vi "set_properties_dialog.vi"(8 "Graph Range Min/Max":T1, 9 "Graph Properties In":T3, 10 "All Properties":T4, 11 "Plot IDs":i32[](array[numeric])) -> (1 "Graph Properties Out":T3, 2 "All Properties Out":T4)   [LabVIEW 2020, in "3DPC_SurfacePlot.xctl"]
uses:
  <vilib>/Native 3D Graph/xcontrol/3DPC_SurfacePlot.xctl
  <vilib>/Native 3D Graph/typedefs/all_non_graph_prop.ctl
  <vilib>/Native 3D Graph/typedefs/prop_plot_all_array.ctl
  <vilib>/Native 3D Graph/typedefs/prop_plot_all.ctl
  <vilib>/Native 3D Graph/typedefs/prop_plot_projection.ctl
  <vilib>/Native 3D Graph/typedefs/prop_plot_surface.ctl
  <vilib>/Native 3D Graph/typedefs/prop_plot_contour.ctl
  <vilib>/Native 3D Graph/typedefs/prop_plot_normal.ctl
  <vilib>/Native 3D Graph/typedefs/prop_plot_point_line.ctl
  <vilib>/Native 3D Graph/typedefs/prop_value_pair_all.ctl
  <vilib>/Native 3D Graph/typedefs/prop_value_pair_1d.ctl
  <vilib>/Native 3D Graph/typedefs/prop_axes_all.ctl
  <vilib>/Native 3D Graph/typedefs/prop_axes_grid.ctl
  <vilib>/Native 3D Graph/typedefs/prop_axes_ticks.ctl
  <vilib>/Native 3D Graph/typedefs/range_cluster.ctl
  <vilib>/Native 3D Graph/typedefs/min_max.ctl
  <vilib>/Native 3D Graph/typedefs/prop_axes_captions.ctl
  <vilib>/Native 3D Graph/typedefs/prop_axes_labels.ctl
  <vilib>/Native 3D Graph/typedefs/prop_axes_autorange.ctl
  <vilib>/Native 3D Graph/typedefs/prop_cursor_all_array.ctl
  <vilib>/Native 3D Graph/typedefs/prop_cursor_point.ctl
  <vilib>/Native 3D Graph/typedefs/prop_cursor_position.ctl
  <vilib>/Native 3D Graph/typedefs/prop_cursor_line.ctl
  <vilib>/Native 3D Graph/typedefs/prop_cursor_plane.ctl
  <vilib>/Native 3D Graph/typedefs/prop_cursor_text.ctl
  <vilib>/Native 3D Graph/typedefs/prop_format.ctl
  <vilib>/Native 3D Graph/typedefs/prop_lighting.ctl
  <vilib>/Native 3D Graph/typedefs/prop_graph.ctl
  <vilib>/Utility/miscctls.llb/LVPointTypeDef.ctl
panel:
  in  "Tab Control":T28(tab)
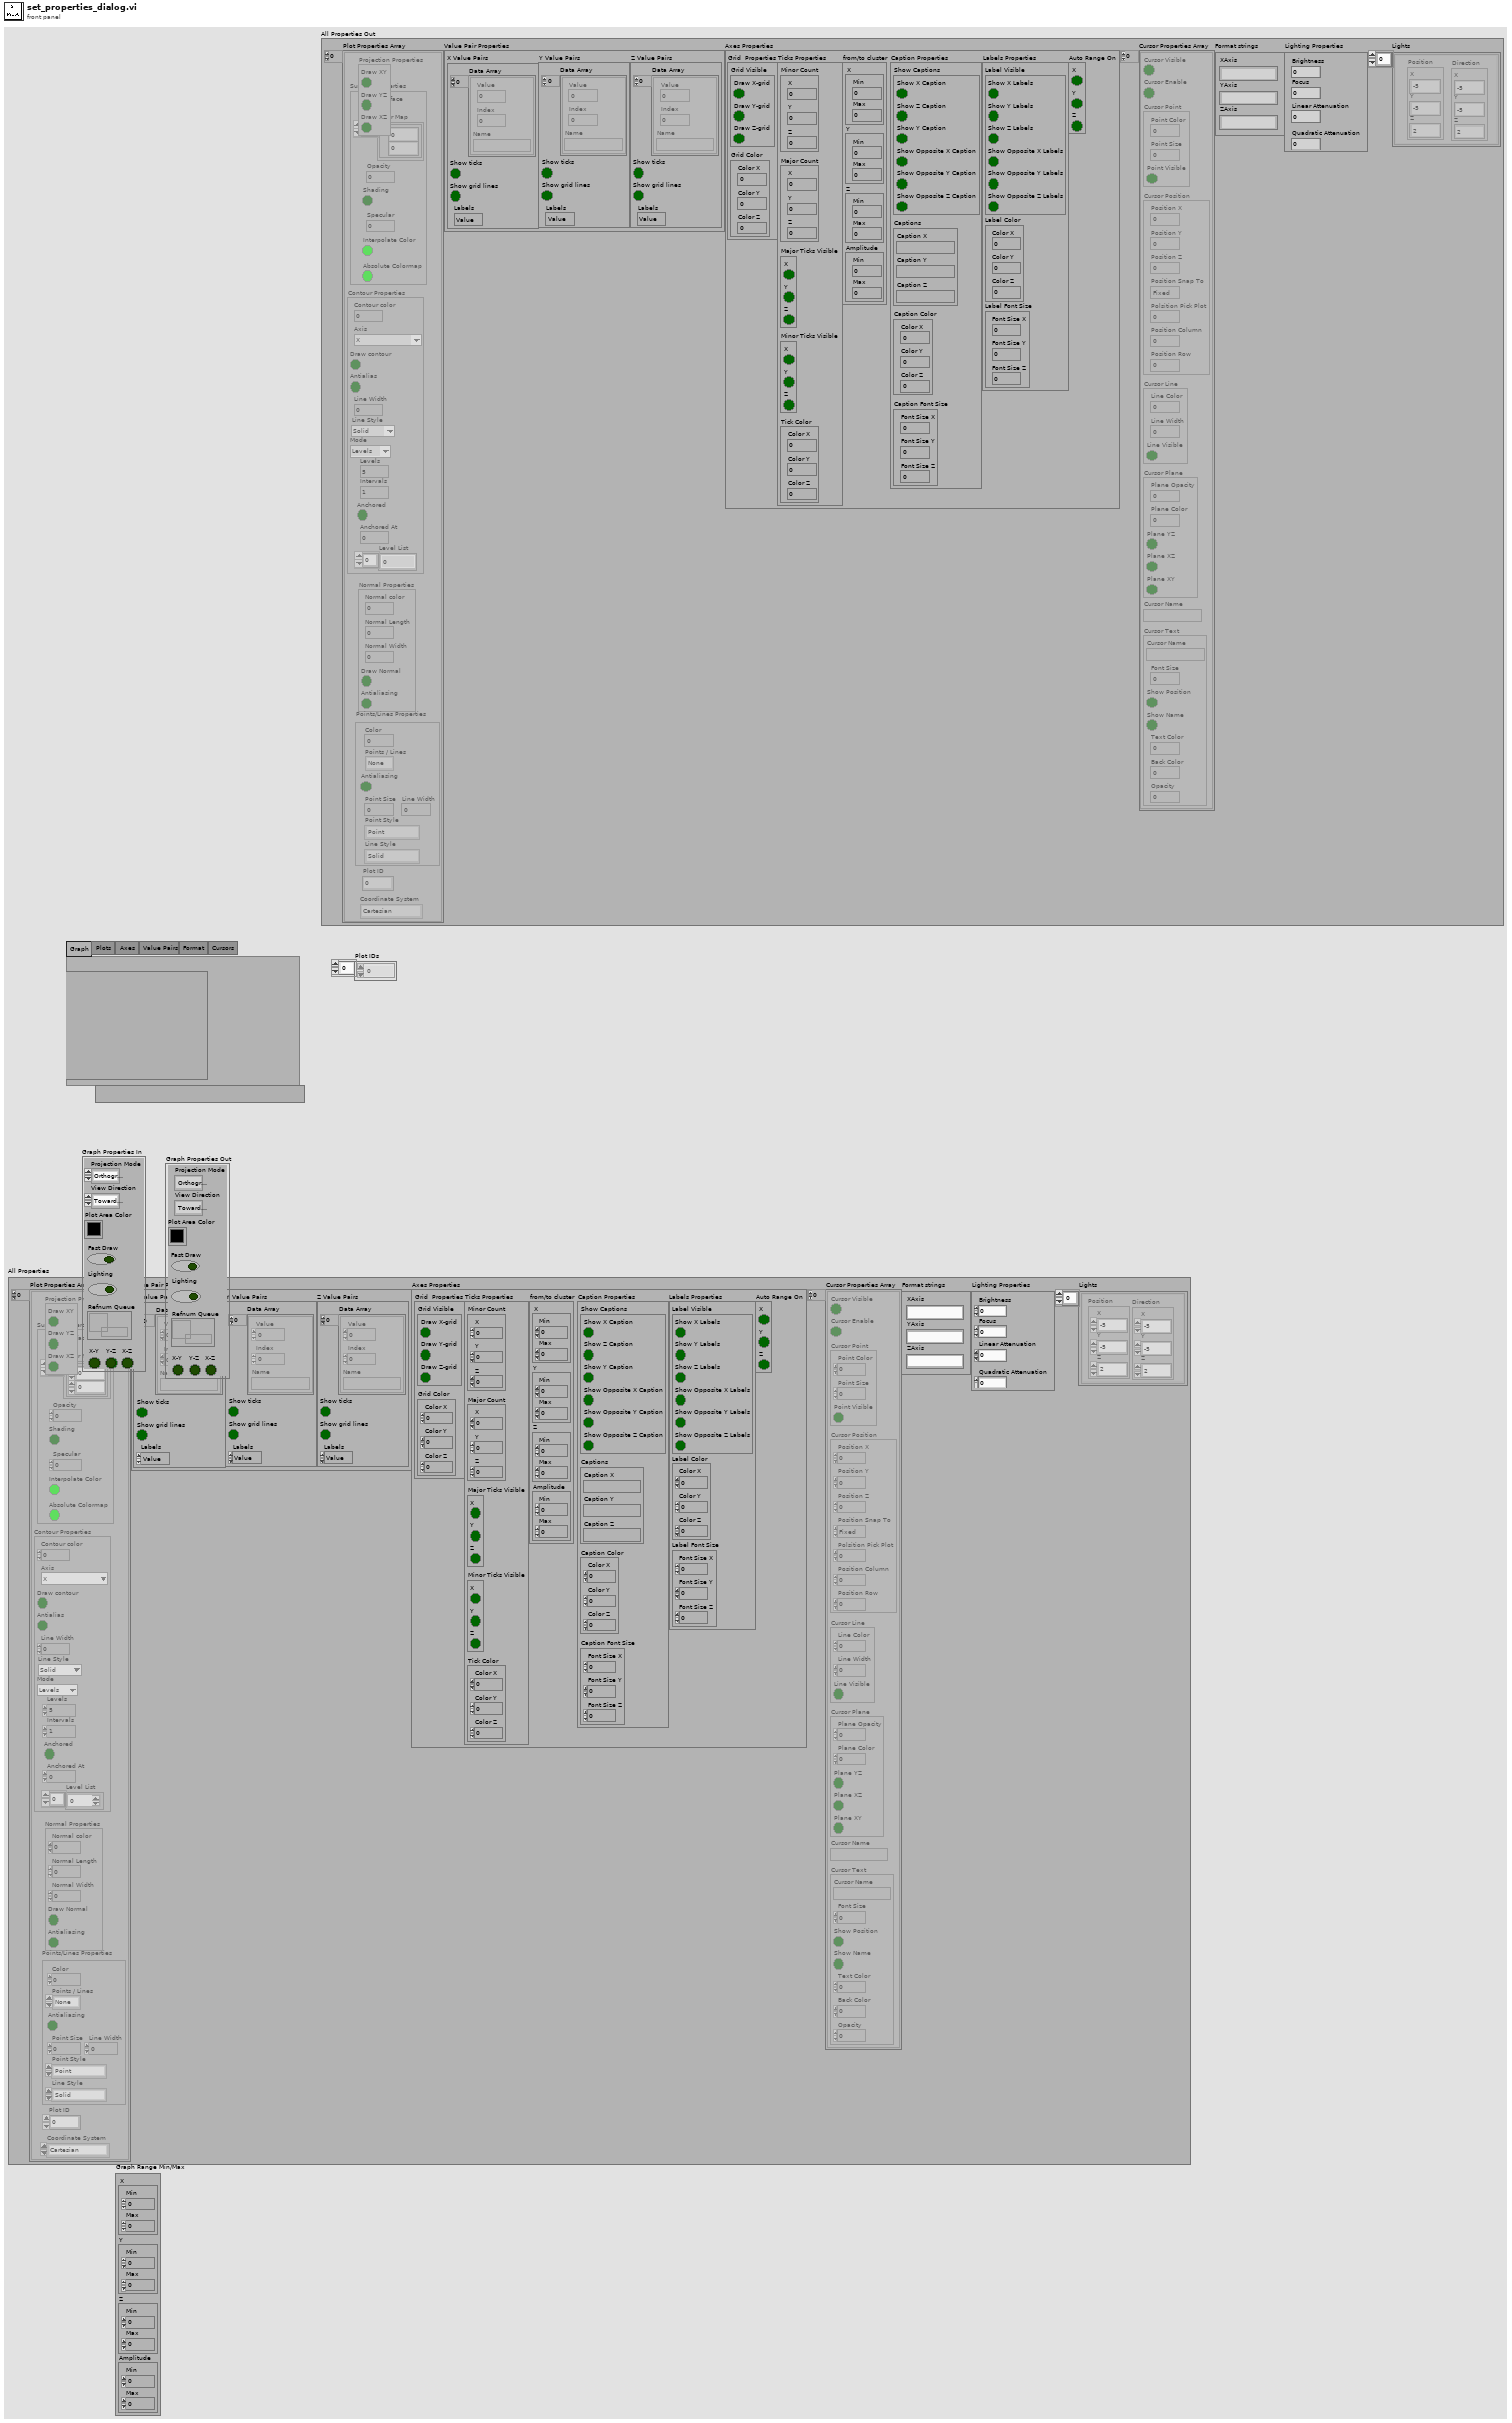
[diagram p1: front panel]
types:
  T1 = typedef "3DPC_SurfacePlot.xctl/range_cluster.ctl" = cluster{"X":T2, "Y":T2, "Z":T2, "Amplitude":T2}
  T2 = typedef "3DPC_SurfacePlot.xctl/min_max.ctl" = cluster{"Min":sgl, "Max":sgl}
  T3 = typedef "3DPC_SurfacePlot.xctl/prop_graph.ctl" = cluster{"Projection Mode":enum16{"Orthographic", "Perspective"}, "View Direction":enum32{"Towards X-Y Plane", "Towards Y-Z Plane", "Towards X-Z Plane", "User Define"}, "Plot Area Color":u32, "Fast Draw":bool, "X-Y":bool, "Y-Z":bool, "X-Z":bool, "Lighting":bool, "Refnum Queue":refnum<queue>}
  T4 = typedef "3DPC_SurfacePlot.xctl/all_non_graph_prop.ctl" = cluster{"Plot Properties Array":T5, "Value Pair Properties":T12, "Axes Properties":T14, "Cursor Properties Array":T20, "Format strings":T26, "Lighting Properties":T27, "Lights":cluster{"Position":cluster{"X":sgl, "Y":sgl, "Z":sgl}, "Direction":cluster{"X":sgl, "Y":sgl, "Z":sgl}}[]}
  T5 = typedef "3DPC_SurfacePlot.xctl/prop_plot_all_array.ctl" = T6[]
  T6 = typedef "3DPC_SurfacePlot.xctl/prop_plot_all.ctl" = cluster{"Projection Properties":T7, "Surface Properties":T8, "Contour Properties":T9, "Normal Properties":T10, "Points/Lines Properties":T11, "Plot ID":i32, "Coordinate System":enum16{"Cartesian", "Cylindrical", "Spherical"}}
  T7 = typedef "3DPC_SurfacePlot.xctl/prop_plot_projection.ctl" = cluster{"Draw XY":bool, "Draw YZ":bool, "Draw XZ":bool}
  T8 = typedef "3DPC_SurfacePlot.xctl/prop_plot_surface.ctl" = cluster{"Draw surface":bool, "Opacity":dbl, "Shading":bool, "Specular":i32, "Color Map":cluster{dbl, u32}[], "Interpolate Color":bool, "Absolute Colormap":bool}
  T9 = typedef "3DPC_SurfacePlot.xctl/prop_plot_contour.ctl" = cluster{"Contour color":u32, "Axis":enum16{"X", "Y", "Z"}, "Draw contour":bool, "Antialias":bool, "Line Width":sgl, "Contour Line Style":enum16{"Solid", "Dash", "Dot", "Dash Dot"}, "Mode":enum16{"Levels", "Intervals", "Level List"}, "Levels":sgl, "Intervals":sgl, "Anchored At":sgl, "Anchored":bool, "Level List":dbl[]}
  T10 = typedef "3DPC_SurfacePlot.xctl/prop_plot_normal.ctl" = cluster{"Normal color":u32, "Normal Length":sgl, "Normal Width":sgl, "Draw Normal":bool, "Antialiasing":bool}
  T11 = typedef "3DPC_SurfacePlot.xctl/prop_plot_point_line.ctl" = cluster{"Color":u32, "Antialiasing":bool, "Point Size":sgl, "Points / Lines":enum16{"None", "Points", "Lines", "Both"}, "Point Style":enum16{"Point", "EmptySquare", "Asterisk", "Diamond", "EmptyCircle", "Circle", "X"}, "Line Style":enum16{"Solid", "Dash", "Dot", "Dash Dot"}, "Line Width":sgl}
  T12 = typedef "3DPC_SurfacePlot.xctl/prop_value_pair_all.ctl" = cluster{"X Value Pairs":cluster{"Data Array":cluster{"Value":sgl, "Index":i32, "Name":string}[], "Show ticks":bool, "Show grid lines":bool, "Labels":enum16{"Value", "None", "Name"}}, "Y Value Pairs":T13, "Z Value Pairs":T13}
  T13 = typedef "3DPC_SurfacePlot.xctl/prop_value_pair_1d.ctl" = cluster{"Data Array":cluster{"Value":sgl, "Index":i32, "Name":string}[], "Show ticks":bool, "Show grid lines":bool, "Labels":enum16{"Value", "None", "Name"}}
  T14 = typedef "3DPC_SurfacePlot.xctl/prop_axes_all.ctl" = cluster{"Grid  Properties":T15, "Ticks Properties":T16, "from/to cluster":T1, "Caption Properties":T17, "Labels Properties":T18, "Auto Range On":T19}
  T15 = typedef "3DPC_SurfacePlot.xctl/prop_axes_grid.ctl" = cluster{"Grid Visible":cluster{"Draw X-grid":bool, "Draw Y-grid":bool, "Draw Z-grid":bool}, "Grid Color":cluster{"Color X":u32, "Color Y":u32, "Color Z":u32}}
  T16 = typedef "3DPC_SurfacePlot.xctl/prop_axes_ticks.ctl" = cluster{"Minor Count":cluster{"X":i32, "Y":i32, "Z":i32}, "Major Count":cluster{"X":i32, "Y":i32, "Z":i32}, "Major Ticks Visible":cluster{"X":bool, "Y":bool, "Z":bool}, "Minor Ticks Visible":cluster{"X":bool, "Y":bool, "Z":bool}, "Tick Color":cluster{"Color X":u32, "Color Y":u32, "Color Z":u32}}
  T17 = typedef "3DPC_SurfacePlot.xctl/prop_axes_captions.ctl" = cluster{"Show Captions":cluster{"Show X Caption":bool, "Show Z Caption":bool, "Show Y Caption":bool, "Show Opposite X Caption":bool, "Show Opposite Y Caption":bool, "Show Opposite Z Caption":bool}, "Captions":cluster{"Caption X":string, "Caption Y":string, "Caption Z":string}, "Caption Color":cluster{"Color X":u32, "Color Y":u32, "Color Z":u32}, "Caption Font Size":cluster{"Font Size X":i16, "Font Size Y":i16, "Font Size Z":i16}}
  T18 = typedef "3DPC_SurfacePlot.xctl/prop_axes_labels.ctl" = cluster{"Label Visible":cluster{"Show X Labels":bool, "Show Y Labels":bool, "Show Z Labels":bool, "Show Opposite X Labels":bool, "Show Opposite Y Labels":bool, "Show Opposite Z Labels":bool}, "Label Color":cluster{"Color X":u32, "Color Y":u32, "Color Z":u32}, "Label Font Size":cluster{"Font Size X":i16, "Font Size Y":i16, "Font Size Z":i16}}
  T19 = typedef "3DPC_SurfacePlot.xctl/prop_axes_autorange.ctl" = cluster{"X":bool, "Y":bool, "Z":bool}
  T20 = typedef "3DPC_SurfacePlot.xctl/prop_cursor_all_array.ctl" = cluster{"Cursor Visible":bool, "Cursor Enable":bool, "Cursor Point":T21, "Cursor Position":T22, "Cursor Line":T23, "Cursor Plane":T24, "Cursor Name":string, "Cursor Text":T25}[]
  T21 = typedef "3DPC_SurfacePlot.xctl/prop_cursor_point.ctl" = cluster{"Point Color":u32, "Point Size":dbl, "Point Visible":bool}
  T22 = typedef "3DPC_SurfacePlot.xctl/prop_cursor_position.ctl" = cluster{"Position X":dbl, "Position Y":dbl, "Position Z":dbl, "Position Snap To":enum16{"Fixed", "Nearest Plot", "Snap to Plot"}, "Polsition Pick Plot":u16, "Position Column":i32, "Position Row":i32}
  T23 = typedef "3DPC_SurfacePlot.xctl/prop_cursor_line.ctl" = cluster{"Line Color":u32, "Line Width":dbl, "Line Visible":bool}
  T24 = typedef "3DPC_SurfacePlot.xctl/prop_cursor_plane.ctl" = cluster{"Plane Opacity":dbl, "Plane Color":u32, "Plane YZ":bool, "Plane XZ":bool, "Plane XY":bool}
  T25 = typedef "3DPC_SurfacePlot.xctl/prop_cursor_text.ctl" = cluster{"Cursor Name":string, "Font Size":i32, "Show Position":bool, "Show Name":bool, "Text Color":u32, "Back Color":u32, "Opacity":dbl}
  T26 = typedef "3DPC_SurfacePlot.xctl/prop_format.ctl" = cluster{"XAxis":string, "YAxis":string, "ZAxis":string}
  T27 = typedef "3DPC_SurfacePlot.xctl/prop_lighting.ctl" = cluster{"Brightness":i32, "Focus":dbl, "Linear Attenuation":dbl, "Quadratic Attenuation":dbl}
  T28 = enum32{"Graph", "Plots ", "Axes ", "Value Pairs", "Format", "Cursors"}
  T29 = typedef "LVPointTypeDef.ctl" = cluster{"Horizontal":i16, "Vertical":i16}
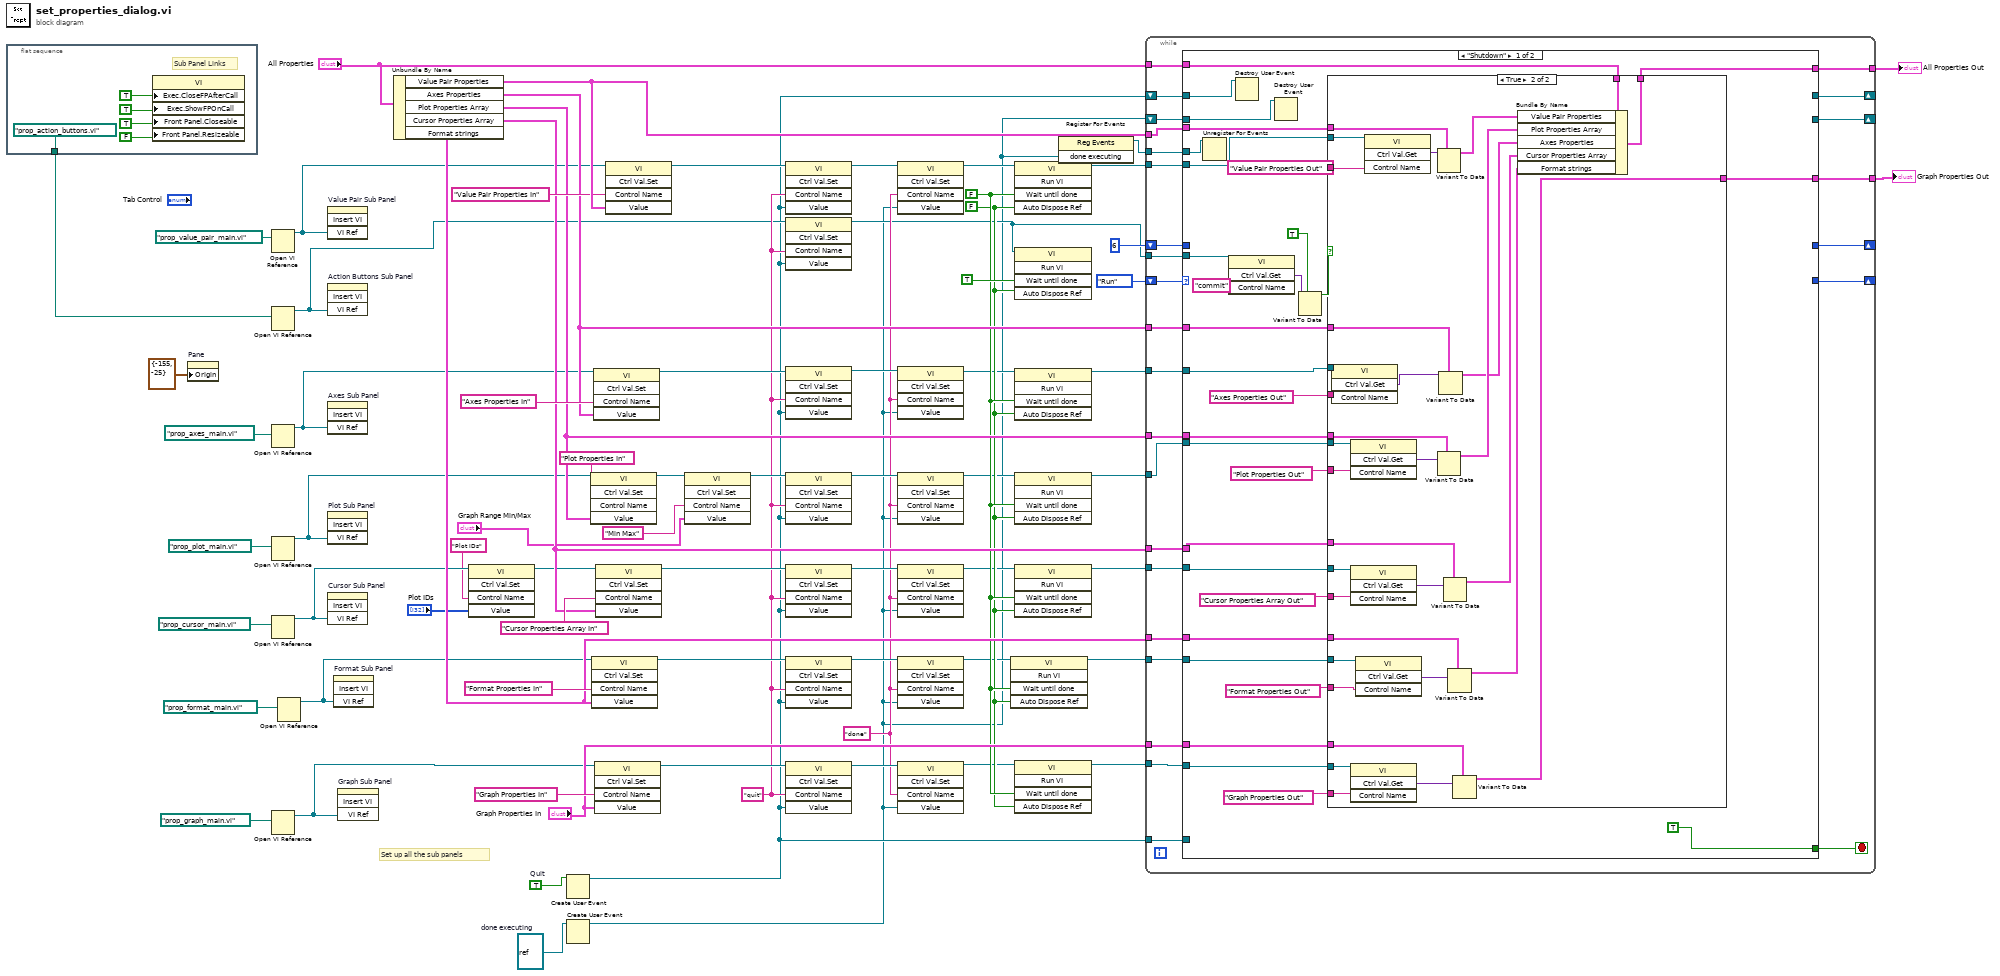
[diagram p0: block diagram]
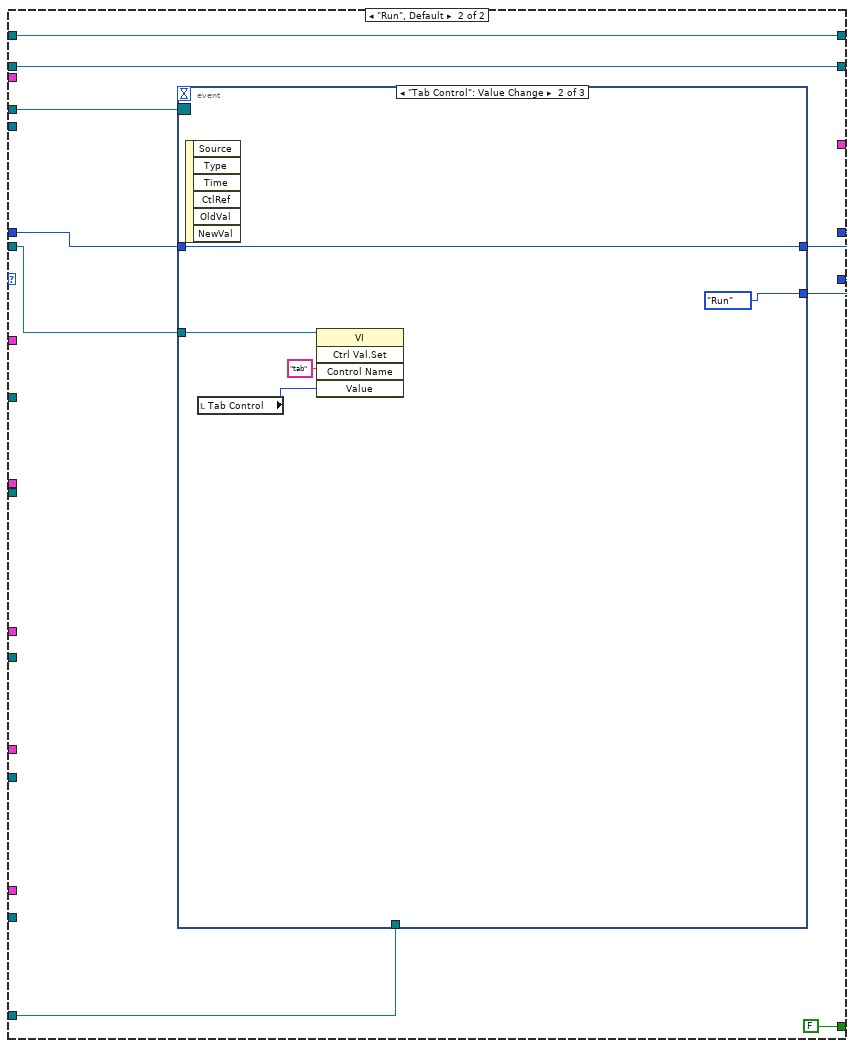
[diagram p3: hidden frame]
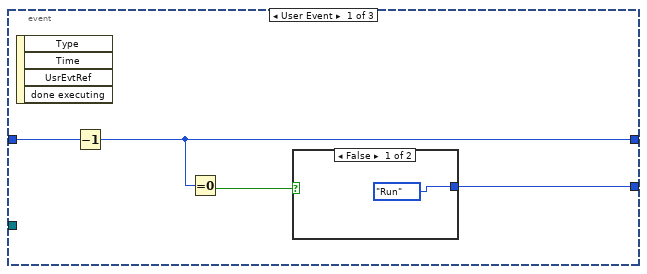
[diagram p4: hidden frame]
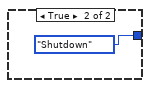
[diagram p5: hidden frame]
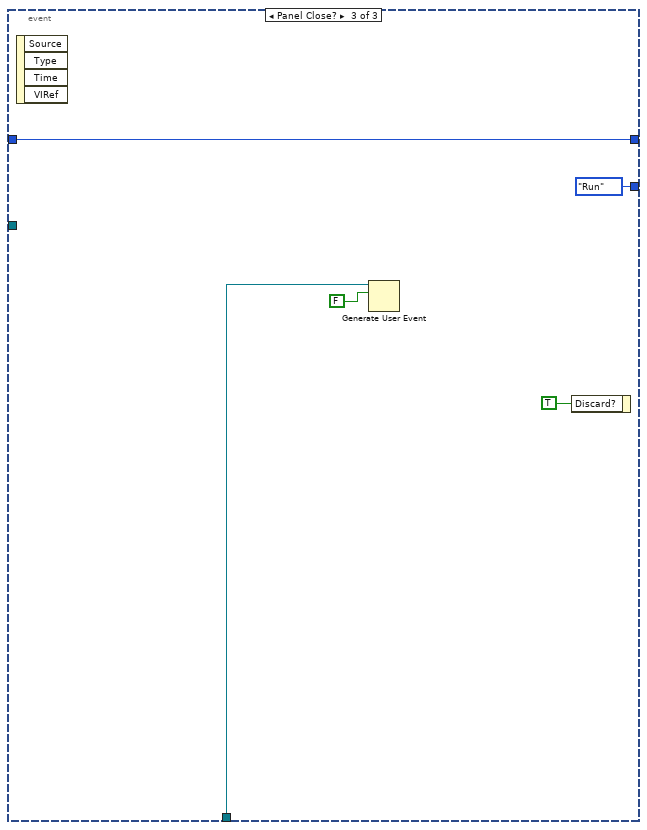
[diagram p6: hidden frame]
diagram:
  w29 = FALSE ("Auto Dispose Reference")
  w30 = FALSE ("Wait Until Done")
  w35 = refnum<vi> refnum  # done executing
  w38 = "done" ("Control Name")
  w39 = "quit" ("Control Name")
  w52 = TRUE  # Quit
  # "Set up all the sub panels"
  n1 = flat-sequence {
    tunnel: [path "prop_action_buttons.vi" ("vi path")] -> w32
    frame #0 {
      # "Sub Panel Links"
      n2 = property class="VI"("Exec.CloseFPAfterCall"=TRUE ("Execution:Close After Call"), "Exec.ShowFPOnCall"=TRUE ("Execution:Show Front Panel On Call"), "Front Panel.Closeable"=TRUE ("Front Panel Window:Closeable"), "Front Panel.Resizeable"=FALSE ("Front Panel Window:Resizeable")) -> ()  [unwired: 2 in, 2 out]
    }
  }
  n3 = property on="Pane" class="Pane"("Origin"=T29 {"Horizontal"=-155, "Vertical"=-25} ("Point")) -> ()  [unwired: 2 in, 2 out]
  n4 = Open VI Reference(vi path=path "prop_value_pair_main.vi") -> (vi reference=w16:refnum<vi>)  [unwired: 1 in, 5 out]
  n5 = Open VI Reference(vi path=w32) -> (vi reference=w15:refnum<vi>)  [unwired: 2 in, 4 out]
  n6 = Open VI Reference(vi path=path "prop_axes_main.vi") -> (vi reference=w14:refnum<vi>)  [unwired: 1 in, 5 out]
  n7 = Open VI Reference(vi path=path "prop_plot_main.vi") -> (vi reference=w5:refnum<vi>)  [unwired: 1 in, 5 out]
  n8 = Open VI Reference(vi path=path "prop_cursor_main.vi") -> (vi reference=w8:refnum<vi>)  [unwired: 1 in, 5 out]
  n9 = Open VI Reference(vi path=path "prop_graph_main.vi") -> (vi reference=w12:refnum<vi>)  [unwired: 1 in, 5 out]
  n10 = Open VI Reference(vi path=path "prop_format_main.vi") -> (vi reference=w13:refnum<vi>)  [unwired: 1 in, 5 out]
  n11 = invoke on="Value Pair Sub Panel" class="SubPnl" method="Insert VI"("VI Ref"=w16) -> ()  [unwired: 3 in, 4 out]
  n12 = invoke on="Action Buttons Sub Panel" class="SubPanel" method="Insert VI"("VI Ref"=w15) -> ()  [unwired: 3 in, 4 out]
  n13 = invoke on="Axes Sub Panel" class="SubPanel" method="Insert VI"("VI Ref"=w14) -> ()  [unwired: 3 in, 4 out]
  n14 = invoke on="Plot Sub Panel" class="SubPanel" method="Insert VI"("VI Ref"=w5) -> ()  [unwired: 3 in, 4 out]
  n15 = invoke on="Cursor Sub Panel" class="SubPnl" method="Insert VI"("VI Ref"=w8) -> ()  [unwired: 3 in, 4 out]
  n16 = invoke on="Format Sub Panel" class="SubPnl" method="Insert VI"("VI Ref"=w13) -> ()  [unwired: 3 in, 4 out]
  n17 = invoke on="Graph Sub Panel" class="SubPnl" method="Insert VI"("VI Ref"=w12) -> ()  [unwired: 3 in, 4 out]
  n18 = Unbundle By Name("All Properties") -> ("Value Pair Properties"=w73:T12, "Axes Properties"=w53:T14, "Plot Properties Array"=w65:T5, "Cursor Properties Array"=w63:T20, "Format strings"=w56:T26)
  n19 = invoke class="VI" method="Ctrl Val.Set"(reference=w8, "Control Name"="Plot IDs", "Value"="Plot IDs") -> (reference out=w9:refnum<vi>)  [unwired: 2 in, 4 out]
  n20 = Create User Event ("Quit")(user event datatype=w52) -> (user event=w2:refnum<user-event>)  [unwired: 1 in, 1 out]
  n21 = Create User Event ("Done")(user event datatype=w35) -> (user event=w1:refnum<user-event>)  [unwired: 1 in, 1 out]
  n22 = invoke class="VI" method="Ctrl Val.Set"(reference=w5, "Control Name"="Plot Properties In", "Value"=w65) -> (reference out=w55:refnum<vi>)  [unwired: 2 in, 4 out]
  n23 = invoke class="VI" method="Ctrl Val.Set"(reference=w13, "Control Name"="Format Properties In", "Value"=w56) -> (reference out=w49:refnum<vi>)  [unwired: 2 in, 4 out]
  n24 = invoke class="VI" method="Ctrl Val.Set"(reference=w14, "Control Name"="Axes Properties In", "Value"=w53) -> (reference out=w43:refnum<vi>)  [unwired: 2 in, 4 out]
  n25 = invoke class="VI" method="Ctrl Val.Set"(reference=w12, "Control Name"="Graph Properties In", "Value"="Graph Properties In") -> (reference out=w51:refnum<vi>)  [unwired: 2 in, 4 out]
  n26 = invoke class="VI" method="Ctrl Val.Set"(reference=w9, "Control Name"="Cursor Properties Array In", "Value"=w63) -> (reference out=w47:refnum<vi>)  [unwired: 2 in, 4 out]
  n27 = invoke class="VI" method="Ctrl Val.Set"(reference=w16, "Control Name"="Value Pair Properties In", "Value"=w73) -> (reference out=w41:refnum<vi>)  [unwired: 2 in, 4 out]
  n28 = invoke class="VI" method="Ctrl Val.Set"(reference=w55, "Control Name"="Min Max", "Value"="Graph Range Min/Max") -> (reference out=w45:refnum<vi>)  [unwired: 2 in, 4 out]
  n29 = invoke class="VI" method="Ctrl Val.Set"(reference=w41, "Control Name"=w39, "Value"=w2) -> (reference out=w40:refnum<vi>)  [unwired: 2 in, 4 out]
  n30 = invoke class="VI" method="Ctrl Val.Set"(reference=w15, "Control Name"=w39, "Value"=w2) -> (reference out=w3:refnum<vi>)  [unwired: 2 in, 4 out]
  n31 = invoke class="VI" method="Ctrl Val.Set"(reference=w43, "Control Name"=w39, "Value"=w2) -> (reference out=w42:refnum<vi>)  [unwired: 2 in, 4 out]
  n32 = invoke class="VI" method="Ctrl Val.Set"(reference=w45, "Control Name"=w39, "Value"=w2) -> (reference out=w44:refnum<vi>)  [unwired: 2 in, 4 out]
  n33 = invoke class="VI" method="Ctrl Val.Set"(reference=w47, "Control Name"=w39, "Value"=w2) -> (reference out=w46:refnum<vi>)  [unwired: 2 in, 4 out]
  n34 = invoke class="VI" method="Ctrl Val.Set"(reference=w49, "Control Name"=w39, "Value"=w2) -> (reference out=w48:refnum<vi>)  [unwired: 2 in, 4 out]
  n35 = invoke class="VI" method="Ctrl Val.Set"(reference=w51, "Control Name"=w39, "Value"=w2) -> (reference out=w50:refnum<vi>)  [unwired: 2 in, 4 out]
  n36 = invoke class="VI" method="Ctrl Val.Set"(reference=w40, "Control Name"=w38, "Value"=w1) -> (reference out=w28:refnum<vi>)  [unwired: 2 in, 4 out]
  n37 = invoke class="VI" method="Ctrl Val.Set"(reference=w42, "Control Name"=w38, "Value"=w1) -> (reference out=w26:refnum<vi>)  [unwired: 2 in, 4 out]
  n38 = invoke class="VI" method="Ctrl Val.Set"(reference=w44, "Control Name"=w38, "Value"=w1) -> (reference out=w24:refnum<vi>)  [unwired: 2 in, 4 out]
  n39 = invoke class="VI" method="Ctrl Val.Set"(reference=w46, "Control Name"=w38, "Value"=w1) -> (reference out=w22:refnum<vi>)  [unwired: 2 in, 4 out]
  n40 = invoke class="VI" method="Ctrl Val.Set"(reference=w48, "Control Name"=w38, "Value"=w1) -> (reference out=w20:refnum<vi>)  [unwired: 2 in, 4 out]
  n41 = invoke class="VI" method="Ctrl Val.Set"(reference=w50, "Control Name"=w38, "Value"=w1) -> (reference out=w18:refnum<vi>)  [unwired: 2 in, 4 out]
  n42 = invoke class="VI" method="Run VI"(reference=w20, "Wait until done"=w30, "Auto Dispose Ref"=w29) -> (reference out=w19:refnum<vi>)  [unwired: 2 in, 4 out]
  n43 = invoke class="VI" method="Run VI"(reference=w28, "Wait until done"=w30, "Auto Dispose Ref"=w29) -> (reference out=w27:refnum<vi>)  [unwired: 2 in, 4 out]
  n44 = invoke class="VI" method="Run VI"(reference=w3, "Wait until done"=TRUE ("Wait Until Done"), "Auto Dispose Ref"=w29) -> ()  [unwired: 2 in, 5 out]
  n45 = invoke class="VI" method="Run VI"(reference=w26, "Wait until done"=w30, "Auto Dispose Ref"=w29) -> (reference out=w25:refnum<vi>)  [unwired: 2 in, 4 out]
  n46 = invoke class="VI" method="Run VI"(reference=w24, "Wait until done"=w30, "Auto Dispose Ref"=w29) -> (reference out=w23:refnum<vi>)  [unwired: 2 in, 4 out]
  n47 = invoke class="VI" method="Run VI"(reference=w22, "Wait until done"=w30, "Auto Dispose Ref"=w29) -> (reference out=w21:refnum<vi>)  [unwired: 2 in, 4 out]
  n48 = invoke class="VI" method="Run VI"(reference=w18, "Wait until done"=w30, "Auto Dispose Ref"=w29) -> (reference out=w17:refnum<vi>)  [unwired: 2 in, 4 out]
  n49 = register-events(w1) -> (reference out=w11:refnum<event-registration>)  [unwired: 2 in, 1 out]
  n50 = while {
    tunnel: "All Properties" -> [w94]
    tunnel: w73 -> [w93]
    tunnel: w53 -> [w87]
    tunnel: w65 -> [w92]
    tunnel: w23 -> [w99]
    tunnel: w25 -> [w100]
    tunnel: w27 -> [w101]
    tunnel: w21 -> [w98]
    tunnel: w63 -> [w91]
    tunnel: w17 -> [w96]
    tunnel: "Graph Properties In" -> [w89]
    tunnel: w19 -> [w97]
    tunnel: w56 -> [w90]
    shift-right: [w102] -> _
    shift-left: enum16{"Run", "Shutdown"}."Run" -> [w105]
    shift-right: [w103] -> _
    shift-left: 6 -> [w104]
    tunnel: [w95] -> w34
    tunnel: [w88] -> w33
    shift-right: [w84] -> _
    shift-left: w1 -> [w85]
    shift-right: [w82] -> _
    shift-left: w2 -> [w83]
    tunnel: w11 -> [w81]
    tunnel: w3 -> [w80]
    tunnel: w2 -> [w79]
    stop <- w86 stop-if-true
    n51 = case shown="\"Shutdown\"" w105 {
      tunnel: w104 -> [_ w178]
      tunnel: [_ w177] -> w103
      tunnel: [_ w176] -> w102
      tunnel: w101 -> [w129 _]
      tunnel: w100 -> [w128 _]
      tunnel: w99 -> [w127 _]
      tunnel: w98 -> [w126 _]
      tunnel: w97 -> [w125 _]
      tunnel: w96 -> [w124 _]
      tunnel: [w123 _] -> w95
      tunnel: w94 -> [w122 _]
      tunnel: w93 -> [w121 _]
      tunnel: w92 -> [w120 _]
      tunnel: w91 -> [w119 _]
      tunnel: w90 -> [w118 _]
      tunnel: w89 -> [w117 _]
      tunnel: [w116 _] -> w88
      tunnel: w87 -> [w115 _]
      tunnel: [TRUE FALSE] -> w86
      tunnel: w85 -> [w112 w175]
      tunnel: [_ w175] -> w84
      tunnel: w83 -> [w113 w174]
      tunnel: [_ w174] -> w82
      tunnel: w81 -> [w111 w172]
      tunnel: w80 -> [w110 w171]
      tunnel: w79 -> [_ w170]
      frame "Shutdown" {
        n52 = Unregister For Events(event registration refnum=w111) -> ()  [unwired: 1 in, 1 out]
        n53 = invoke class="VI" method="Ctrl Val.Get"(reference=w110, "Control Name"="commit") -> ("Get Control Value Variant"=w108:variant)  [unwired: 2 in, 3 out]
        n54 = Destroy User Event(user event=w113) -> ()  [unwired: 1 in, 1 out]
        n55 = Destroy User Event(user event=w112) -> ()  [unwired: 1 in, 1 out]
        n56 = Variant To Data(type=TRUE, Variant=w108) -> (data=w106:bool)  [unwired: 1 in, 1 out]
        n57 = case shown="True" w106 {
          tunnel: "Value Pair Properties Out" ("Control Name") -> [_ w167]
          tunnel: "Plot Properties Out" ("Control Name") -> [_ w166]
          tunnel: "Cursor Properties Array Out" ("Control Name") -> [_ w161]
          tunnel: "Graph Properties Out" ("Control Name") -> [_ w159]
          tunnel: "Axes Properties Out" ("Control Name") -> [_ w157]
          tunnel: "Format Properties Out" ("Control Name") -> [_ w155]
          tunnel: w129 -> [_ w152]
          tunnel: w128 -> [_ w151]
          tunnel: w127 -> [_ w150]
          tunnel: w126 -> [_ w149]
          tunnel: w125 -> [_ w148]
          tunnel: w124 -> [_ w147]
          tunnel: [w137 w146] -> w123
          tunnel: w122 -> [w137 w145]
          tunnel: w121 -> [_ w144]
          tunnel: w120 -> [_ w143]
          tunnel: w119 -> [_ w142]
          tunnel: w118 -> [_ w141]
          tunnel: w117 -> [w136 w140]
          tunnel: [w136 w139] -> w116
          tunnel: w115 -> [_ w138]
          frame False {
          }
          frame True {
            n58 = invoke class="VI" method="Ctrl Val.Get"(reference=w151, "Control Name"=w157) -> ("Get Control Value Variant"=w156:variant)  [unwired: 2 in, 3 out]
            n59 = invoke class="VI" method="Ctrl Val.Get"(reference=w150, "Control Name"=w166) -> ("Get Control Value Variant"=w165:variant)  [unwired: 2 in, 3 out]
            n60 = invoke class="VI" method="Ctrl Val.Get"(reference=w149, "Control Name"=w161) -> ("Get Control Value Variant"=w162:variant)  [unwired: 2 in, 3 out]
            n61 = invoke class="VI" method="Ctrl Val.Get"(reference=w147, "Control Name"=w159) -> ("Get Control Value Variant"=w158:variant)  [unwired: 2 in, 3 out]
            n62 = invoke class="VI" method="Ctrl Val.Get"(reference=w148, "Control Name"=w155) -> ("Get Control Value Variant"=w154:variant)  [unwired: 2 in, 3 out]
            n63 = invoke class="VI" method="Ctrl Val.Get"(reference=w152, "Control Name"=w167) -> ("Get Control Value Variant"=w164:variant)  [unwired: 2 in, 3 out]
            n64 = Variant To Data(type=w144, Variant=w164) -> (data=w168:T12)  [unwired: 1 in, 1 out]
            n65 = Variant To Data(type=w143, Variant=w165) -> (data=w169:T5)  [unwired: 1 in, 1 out]
            n66 = Variant To Data(type=w138, Variant=w156) -> (data=w163:T14)  [unwired: 1 in, 1 out]
            n67 = Variant To Data(type=w142, Variant=w162) -> (data=w160:T20)  [unwired: 1 in, 1 out]
            n68 = Variant To Data(type=w141, Variant=w154) -> (data=w153:T26)  [unwired: 1 in, 1 out]
            n69 = Variant To Data(type=w140, Variant=w158) -> (data=w139:T3)  [unwired: 1 in, 1 out]
            n70 = Bundle By Name(cluster=w145, "Value Pair Properties"=w168, "Plot Properties Array"=w169, "Axes Properties"=w163, "Cursor Properties Array"=w160, "Format strings"=w153) -> (w146:T4)
          }
        }
      }
      frame "Run", Default {
        n71 = event shown="[1] \"Tab Control\": Value Change" {
          selector: w172 -> [_ _ _]
          dyn-events: _ -> [_ _ _]
          timeout: _ -> [_ _ _]
          tunnel: w178 -> [w182 w186 w191]
          tunnel: [w181 w186 w191] -> w177
          tunnel: [w179 enum16{"Run", "Shutdown"}."Run" enum16{"Run", "Shutdown"}."Run"] -> w176
          tunnel: w171 -> [_ w189 _]
          tunnel: w170 -> [_ _ w192]
          event User Event {
            n72 = event-data() -> ()  [unwired: 5 out]
            n73 = Decrement(x=w182) -> (x-1=w181:i32)
            n74 = Equal To 0?(x=w181) -> (x = 0?=w180:bool)
            n75 = case shown="False" w180 {
              tunnel: [enum16{"Run", "Shutdown"}."Run" enum16{"Run", "Shutdown"}."Shutdown"] -> w179
              frame False {
              }
              frame True {
              }
            }
          }
          event "Tab Control": Value Change {
            n76 = event-data() -> ()  [unwired: 7 out]
            n77 = local read "Tab Control"() -> (w187:T28)
            n78 = invoke class="VI" method="Ctrl Val.Set"(reference=w189, "Control Name"="tab", "Value"=w187) -> ()  [unwired: 2 in, 5 out]
          }
          event Panel Close? {
            n79 = event-data() -> ()  [unwired: 5 out]
            n80 = Generate User Event(user event=w192, event data cluster=FALSE ("event data")) -> ()  [unwired: 2 in, 2 out]
            n81 = event-data("Discard?"=TRUE) -> ()  [unwired: 1 in, 1 out]
          }
        }
      }
    }
  }
  "All Properties Out" <- w34
  "Graph Properties Out" <- w33
